vi "connect.vi"(8 "error in (no error)":errorcluster, 10 "IP":string="192.109.209.229", 11 "DLLPath":path) -> (0 "error out":errorcluster, 1 "Device Code":i32, 2 "TDeviceInfo":T1 {"nb of slots" min=5 max=7}, 3 "ID Out":i32, 4 "ECLibDLLPath":path)   [LabVIEW 2022 SP3, in "EClib functions.lvlib"]
doc: "This VI establishes the IP connection between the computer and the instrument selected."
uses:
  EClib functions.lvlib
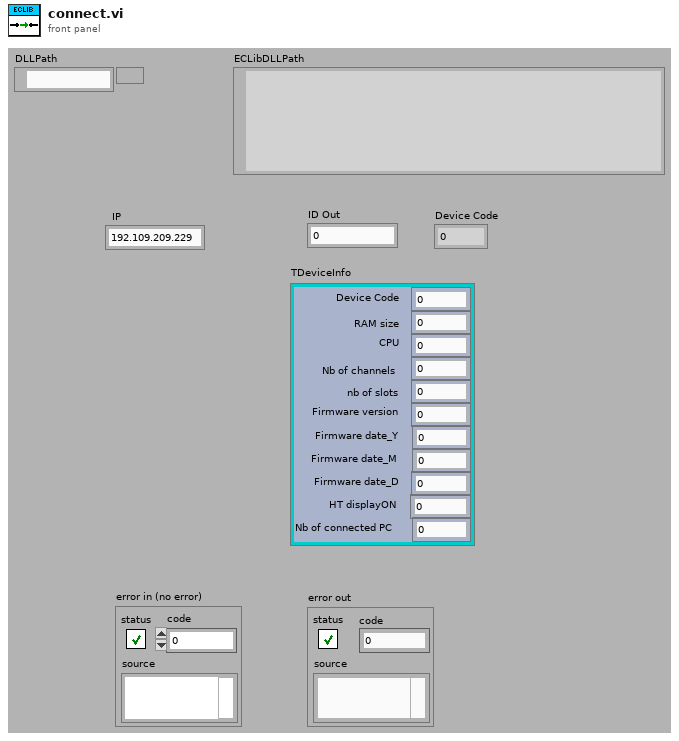
[diagram p1: front panel]
types:
  T1 = cluster{"Device Code":i32, "RAM size":i32, "CPU":i32, "Nb of channels":i32, "nb of slots":i32, "Firmware version":i32, "Firmware date_Y":i32, "Firmware date_M":i32, "Firmware date_D":i32, "HT displayON":i32, "Nb of connected PC":i32}
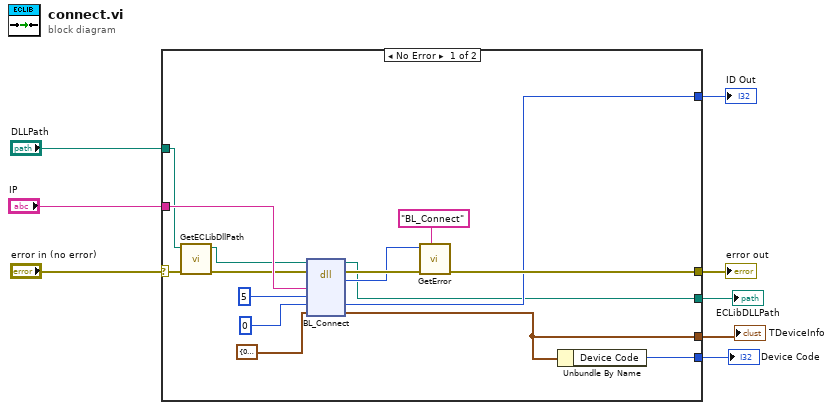
[diagram p0: block diagram]
diagram:
  n1 = case shown="No Error" "error in (no error)" {
    selector: "error in (no error)" -> [w22 w25]
    tunnel: [w16 w25] -> w7
    tunnel: "IP" -> [w21 _]
    tunnel: [w20 _] -> w5
    tunnel: [w19 _] -> w4
    tunnel: [w12 _] -> w3
    tunnel: [w10 _] -> w2
    tunnel: "DLLPath" -> [w9 _]
    frame No Error {
      n2 = call "GetECLibDllPath.vi"("error in (no error)"=w22, "DLLPath"=w9) -> ("error out"=w18:errorcluster, "ECLibDLLPath"=w11:path)  [unwired: 8 in]
      n3 = dll-call lib="?" fn="BL_Connect"(path in=w11, error in=w18, "arg1"=w21, "arg2"=u8 5, "arg3"=0, "arg4"=T1 {"Device Code"=0, "RAM size"=0, "CPU"=0, "Nb of channels"=0, "nb of slots"=0, "Firmware version"=0, "Firmware date_Y"=0, "Firmware date_M"=0, "Firmware date_D"=0, "HT displayON"=0, "Nb of connected PC"=0} ("TDeviceINfo")) -> (path out=w10:path, error out=w17:errorcluster, "return type"=w15:i32, "arg3"=w12:i32, "arg4"=w19:T1)  [unwired: 3 in]
      n4 = call "GetError.vi"("DLLFunction"="BL_Connect", "error in"=w17, "code"=w15) -> ("error out"=w16:errorcluster)  [unwired: 8 in]
      n5 = Unbundle By Name(w19) -> ("Device Code"=w20:i32)
    }
    frame Error {
    }
  }
  "error out" <- w7
  "Device Code" <- w5
  "TDeviceInfo" <- w4
  "ID Out" <- w3
  "ECLibDLLPath" <- w2
